vi "Write Data.vi"(8 "error in (no error)":errorcluster, 9 "Publication Time":timestamp, 10 "Value":variant, 11 "EventTransport In":refnum<class "EventTransport.lvclass">) -> (0 "error out":errorcluster, 3 "EventTransport Out":refnum<class "EventTransport.lvclass">)   [LabVIEW 2020, in "EventTransport.lvclass"]
doc: "<License>\nCopyright © 2017 Composed Systems, LLC | All rights reserved\nwww.composed.io\n\nAuthor: Ethan Stern <ethan.stern@composed.io>\n\nThis software is provided \"AS IS\" WITHOUT WARRANTIES, either express or implied, AND IS FOR EDUCATIONAL PURPOSES ONLY.\n</License>"
uses:
  <vilib>/gpm_packages/@cs/transport/Source/Concrete/EventTransport/EventTransport.lvclass
  <vilib>/gpm_packages/@cs/transport/Source/Concrete/EventTransport/EventTransport.lvclass/EventTransport.ctl
  <vilib>/Utility/error.llb/Error Cluster From Error Code.vi
  <vilib>/ErrorRing/Error Ring.xnode
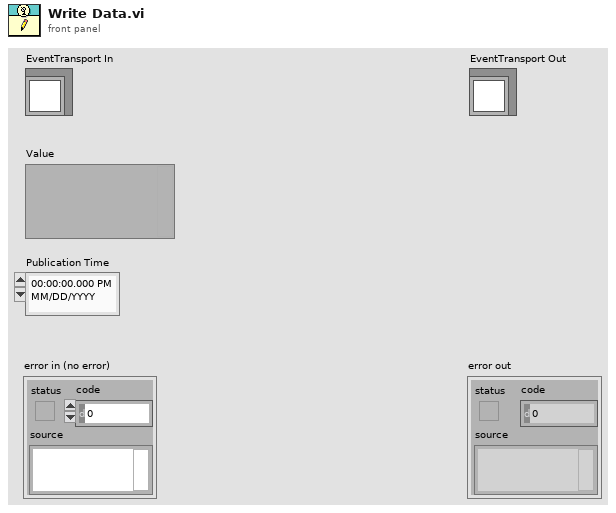
[diagram p1: front panel]
types:
  T1 = typedef "usereventprio.ctl" = enum32{"high priority", "normal priority"}
  T2 = cluster{"Value":variant, "Publication Time":timestamp}
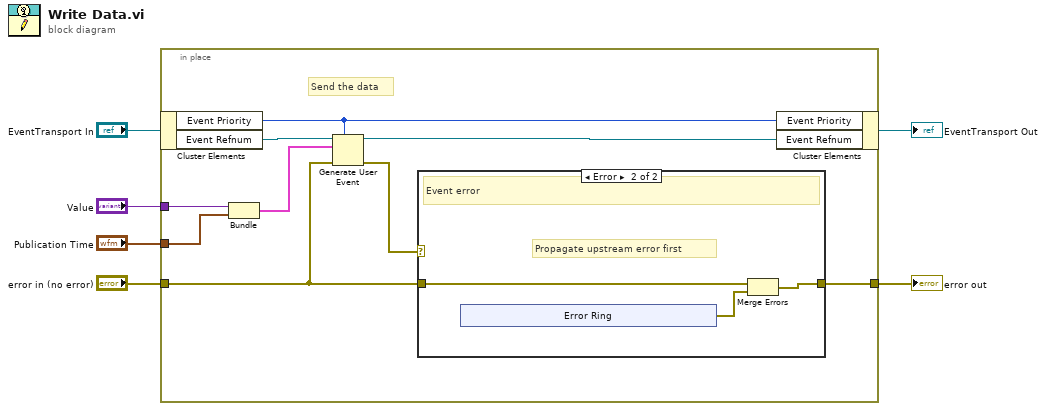
[diagram p0: block diagram]
diagram:
  n1 = in-place {
    in-place-border: "error in (no error)" -> [w8]
    in-place-border: "Value" -> [w15]
    in-place-border: "Publication Time" -> [w14]
    in-place-border: [w9] -> w1
    # "Send the data"
    n2 = in-place-cluster #1("EventTransport In") -> ("Event Priority"=w10:T1, "Event Refnum"=w12:refnum<user-event>)
    n3 = Bundle("Value"=w15, "Publication Time"=w14) -> (w13:T2)  [unwired: 1 in]
    n4 = Generate User Event(priority (normal)=w10, user event=w12, event data cluster=w13, error in=w8) -> (user event out=w11:refnum<user-event>, error out=w7:errorcluster)
    n5 = case shown="Error" w7 {
      selector: w7 -> [w16 _]
      tunnel: [w16 w19] -> w9
      tunnel: w8 -> [_ w17]
      frame No Error {
        # "Things seem normal"
      }
      frame Error {
        # "Propagate upstream error first"
        # "Event error"
        n6 = xnode "Error Ring"() -> ("error out"=w18:errorcluster)
        n7 = Merge Errors(w17, w18) -> (w19:errorcluster)
      }
    }
    n8 = in-place-cluster #1("Event Priority"=w10, "Event Refnum"=w11) -> (→"EventTransport Out":refnum<class "EventTransport.lvclass">)
  }
  "error out" <- w1
